vi "Areotech calc move timeout.vi"(9 "Numeric in":i32, 10 "Position":dbl, 11 "AerotechStage in":refnum<class "AerotechStage.lvclass">) -> (2 "Numeric out":dbl, 3 "Value":dbl)   [LabVIEW 2013, in "AerotechStage.lvclass"]
uses:
  AerotechStage.lvclass
  AerotechStage.lvclass/AerotechStage.ctl
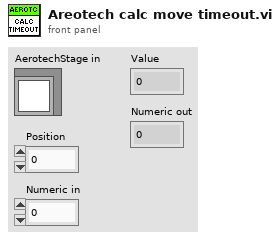
[diagram p1: front panel]
types:
  T1 = cluster{"Axis1":cluster{"Value":dbl, "Min":dbl, "Max":dbl, "StepSize":dbl, "Tolerance":dbl, "ValueActual":dbl}, "Axis2":cluster{"Value":dbl, "Min":dbl, "Max":dbl, "StepSize":dbl, "Tolerance":dbl, "ValueActual":dbl}, "Axis3":cluster{"Value":dbl, "Min":dbl, "Max":dbl, "StepSize":dbl, "Tolerance":dbl, "ValueActual":dbl}}
  T2 = cluster{"Value":dbl, "Min":dbl, "Max":dbl, "StepSize":dbl, "Tolerance":dbl, "ValueActual":dbl}[]
  T3 = cluster{"Value":dbl, "Min":dbl, "Max":dbl, "StepSize":dbl, "Tolerance":dbl, "ValueActual":dbl}
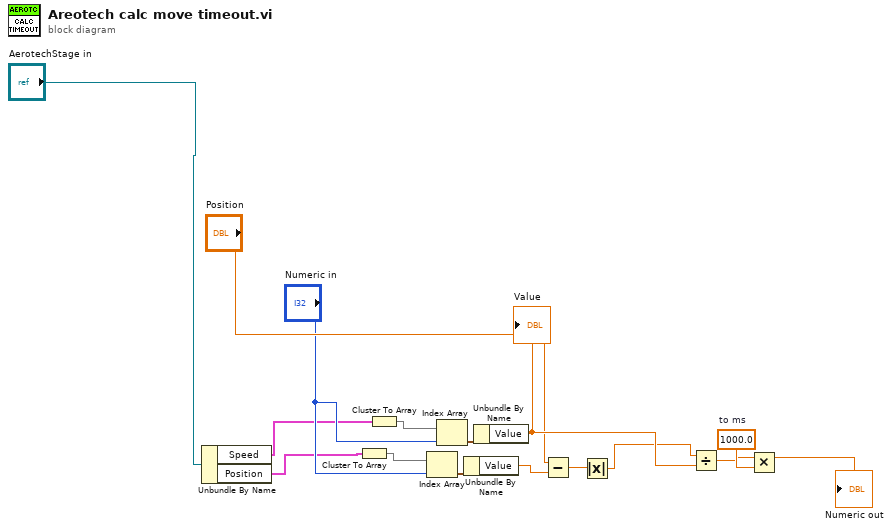
[diagram p0: block diagram]
diagram:
  w16 = 1000.0  # to ms
  n1 = Unbundle By Name("AerotechStage in") -> ("Speed"=w7:T1, "Position"=w4:T1)
  n2 = Cluster To Array(cluster=w4) -> (array=w2:T2)
  n3 = Cluster To Array(cluster=w7) -> (array=w5:T2)
  n4 = Index Array(array=w2, index="Numeric in") -> (element=w1:T3)
  n5 = Index Array(array=w5, index="Numeric in") -> (element=w6:T3)
  n6 = Unbundle By Name(w1) -> ("Value"=w10:dbl)
  n7 = Unbundle By Name(w6) -> ("Value"=w13:dbl)
  "Value" <- w13
  n8 = Subtract(x="Position", y=w10) -> (x-y=w11:dbl)
  n9 = Absolute Value(x=w11) -> (abs(x)=w12:dbl)
  n10 = Divide(x=w12, y=w13) -> (x/y=w14:dbl)
  n11 = Multiply(x=w14, y=w16) -> (x*y=→"Numeric out":dbl)
